vi "SetMode.vi"(0 "VISA resource name":refnum<visa-resource-name>, 5 "Combo Box":string(combo), 11 "error in (no error)":errorcluster) -> (4 "VISA resource name out":refnum<visa-resource-name>, 15 "error out":errorcluster)   [LabVIEW 2024, in "EFmeter.lvlib"]
uses:
  EFmeter.lvlib
panel:
  out "Error Message":string
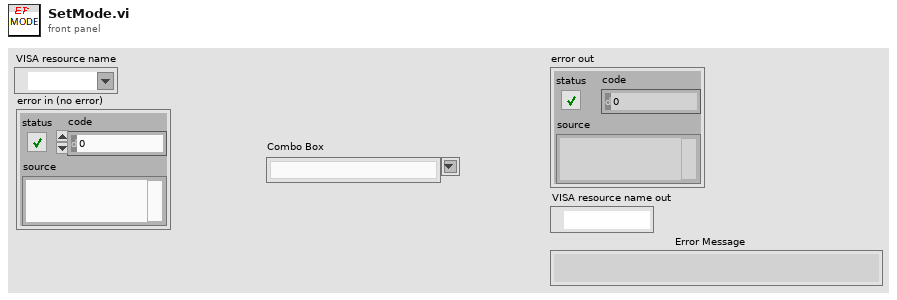
[diagram p1: front panel]
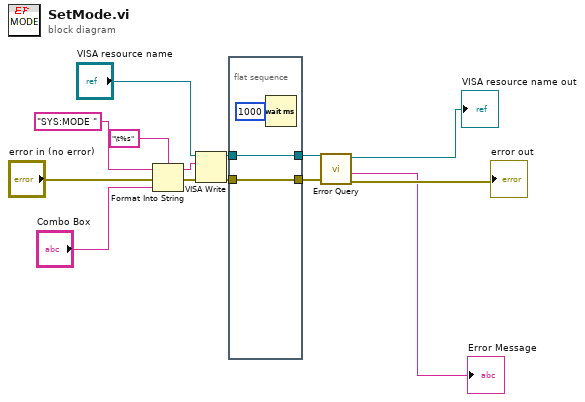
[diagram p0: block diagram]
diagram:
  n1 = Format Into String(format string="\t%s", initial string="SYS:MODE ", error in="error in (no error)", "Combo Box") -> (resulting string=w8:string, error out=w12:errorcluster)
  n2 = VISA Write(VISA resource name="VISA resource name", write buffer=w8, error in (no error)=w12) -> (VISA resource name out=w4:refnum<visa-resource-name>, error out=w2:errorcluster)  [unwired: 1 out]
  n3 = flat-sequence {
    tunnel: w4 -> [w17]
    tunnel: [w17] -> w3
    tunnel: [w16] -> w1
    tunnel: w2 -> [w16]
    frame #0 {
      n4 = Wait (ms)(milliseconds to wait=u32 1000) -> ()  [unwired: 1 out]
    }
  }
  n5 = call "Error Query.vi"("error in (no error)"=w1, "VISA resource name"=w3) -> ("error out"=→"error out":errorcluster, "Error Message"=→"Error Message":string, "VISA resource name out"=→"VISA resource name out":refnum<visa-resource-name>)  [unwired: 6 in, 1 out]
